vi "rus fit - read freq file.vi"(4 "temperature points IN":dbl[](array[numeric])=array[7043 elements], 5 "right":dbl=10069.29999999702, 6 "time points IN":dbl[](array[numeric])=array[7043 elements], 7 "left":dbl, 8 "file path":path=path "\\\\rus-one\\newdata/data/Ultrasound/Experiment/ProbeTest/Probe10/Hg1201-6-C185-550Cair-3c-83K/sweep3/9w/3366_a.dat", 9 "attenuation points IN":dbl[](array[numeric])=array[7043 elements], 10 "frequency points IN":dbl[](array[numeric])=array[7043 elements], 11 "lorentzian points IN":T1[](array[typedef])=array[7043 elements] {"lorentzian"."z∞ (V)" format="%#_4p"; "lorentzian"."Q" format="%#_4p"; "lorentzian"."φ (rad)" format="%#_3p"; "lorentzian"."Γ (Hz)" format="%#_5p"; "lorentzian"."ω (Hz)" format="%#_9p"; "lorentzian"."A (VHz)" format="%#_3p"}) -> (0 "format version":string="A1", 1 "attenuation points OUT":dbl[](array[numeric]), 2 "frequency points OUT":dbl[](array[numeric]), 3 "lorentzian points OUT":T1[](array[typedef]) {"lorentzian"."z∞ (V)" format="%#_4p"; "lorentzian"."Q" format="%#_4p"; "lorentzian"."φ (rad)" format="%#_3p"; "lorentzian"."Γ (Hz)" format="%#_5p"; "lorentzian"."ω (Hz)" format="%#_9p"; "lorentzian"."A (VHz)" format="%#_3p"})   [LabVIEW 2021]
uses:
  temperature sweep point.ctl
  lorentzian.ctl
  circle corners.ctl
  <vilib>/Utility/file.llb/Read From Spreadsheet File (string).vi
  <vilib>/regexp/Match Regular Expression.xnode
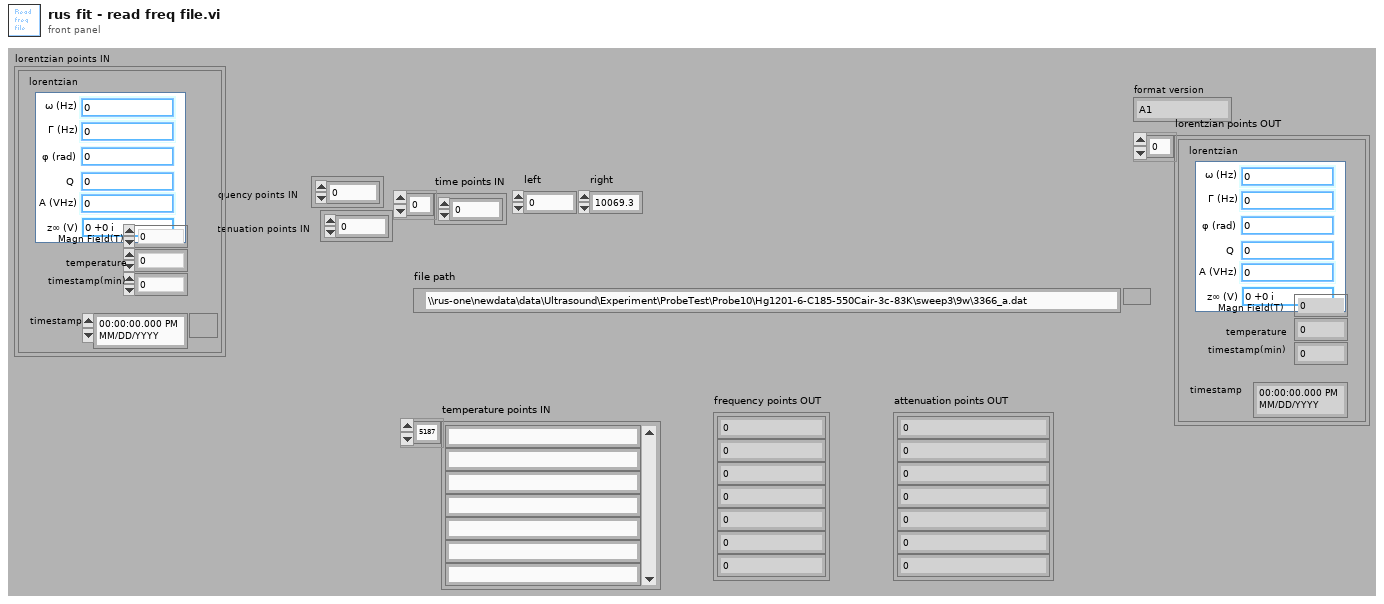
[diagram p1: front panel]
types:
  T1 = typedef "temperature sweep point.ctl" = cluster{"temperature":dbl, "lorentzian":T2, "timestamp(min)":dbl, "timestamp":timestamp, "Magn Field(T)":dbl}
  T2 = typedef "lorentzian.ctl" = cluster{"A (VHz)":dbl, "ω (Hz)":dbl, "Γ (Hz)":dbl, "φ (rad)":dbl, "Q":dbl, "Norm  Ampl":dbl, "z∞ (V)":cdb, "4corners":T3}
  T3 = typedef "circle corners.ctl" = cluster{"z (-pi/2)":cdb, "z(inf)":cdb, "z (pi/2)":cdb, "z center":cdb, "z(0)":cdb, "radius":dbl}
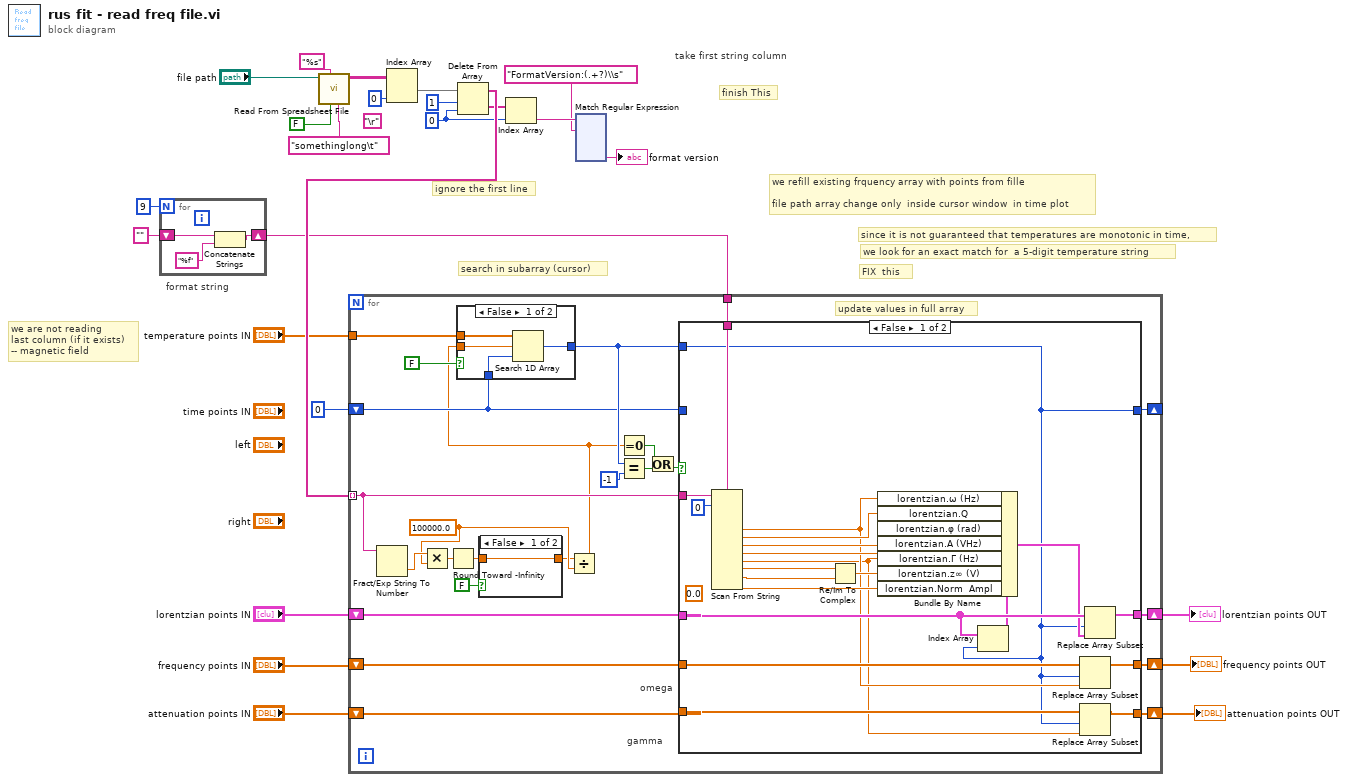
[diagram p0: block diagram]
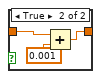
[diagram p2: hidden frame]
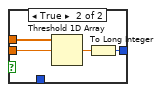
[diagram p3: hidden frame]
diagram:
  w16 = 0 ("index")
  (unwired) "\r"
  # "we are not reading \nlast column (if it exists) \n-- magnetic field"
  # "search in subarray (cursor)"
  # "format string"
  # "since it is not guaranteed that temperatures are monotonic in time,"
  # "we look for an exact match for  a 5-digit temperature string"
  # "FIX  this"
  # "finish This"
  # "take first string column"
  # "we refill existing frquency array with points from fille\n\nfile path array change only  inside cursor window  in time plot"
  # "ignore the first line"
  n1 = for {
    N: 9 -> [_]
    shift-right: [w27] -> w3
    shift-left: "" ("input string") -> [w26]
    n2 = Concatenate Strings(w26, "%f" ("input string")) -> (w27:string)
  }
  n3 = call-poly <vilib>:"Read From Spreadsheet File.vi"("delimiter (\\t)"="somethinglong\t" ("delimiter (\\t)"), "transpose (no:F)"=FALSE ("append to file? (new file:F)"), "format (%s)"="%s", "file path (dialog if empty)"="file path") -> ("all rows"=w22:string[][])  [unwired: 3 in, 4 out]
  n4 = Index Array(array=w22, index (col)=0 ("disabled index (col)")) -> (element=w20:string[])  [unwired: 1 in]
  n5 = Delete From Array(array=w20, length=1, index=w16) -> (deleted portion=w17:string[], array with subset deleted=w18:string[])
  n6 = for {
    shift-right: [w48] -> w9
    shift-left: "attenuation points IN" -> [w47]
    tunnel: w18 -> [w40] mode=indexing
    shift-right: [w51] -> w11
    shift-left: "lorentzian points IN" -> [w52]
    shift-right: [w49] -> w10
    shift-left: "frequency points IN" -> [w50]
    tunnel: "temperature points IN" -> [w41]
    tunnel: w3 -> [w38]
    shift-right: [w37] -> _
    shift-left: 0 -> [w36]
    w33 = 100000.0 ("y")
    # "omega"
    # "gamma"
    # "update values in full array"
    n7 = Fract/Exp String To Number(string=w40) -> (number=w34:dbl)  [unwired: 3 in, 1 out]
    n8 = Multiply(x=w34, y=w33) -> (x*y=w35:dbl)
    n9 = Round Toward -Infinity(1:w35) -> (0:w32:dbl)
    n10 = case shown="False" FALSE {
      tunnel: w32 -> [w53 w55]
      tunnel: [w53 w54] -> w31
      frame False {
      }
      frame True {
        n11 = Add(x=w55, y=0.001) -> (x+y=w54:dbl)
      }
    }
    n12 = Divide(x=w31, y=w33) -> (x/y=w30:dbl)
    n13 = case shown="False" FALSE {
      tunnel: w41 -> [w60 w64]
      tunnel: w30 -> [w59 w61]
      tunnel: [w58 w62] -> w39
      tunnel: w36 -> [w57 _]
      frame False {
        n14 = Search 1D Array(1D array=w60, element=w59, start index (0)=w57) -> (index of element=w58:i32)
      }
      frame True {
        n15 = Threshold 1D Array(2:w61, 3:w64) -> (0:w63:dbl)  [unwired: 1 in]
        n16 = To Long Integer(number=w63) -> (32bit integer=w62:i32)
      }
    }
    n17 = Equal To 0?(x=w30) -> (x = 0?=w46:bool)
    n18 = Equal?(x=w39, y=-1) -> (x = y?=w45:bool)
    n19 = Or(x=w46, y=w45) -> (x .or. y?=w42:bool)
    n20 = case shown="False" w42 {
      tunnel: w52 -> [w80 w89]
      tunnel: [w85 w89] -> w51
      tunnel: w50 -> [w84 w88]
      tunnel: [w83 w88] -> w49
      tunnel: [w82 w87] -> w48
      tunnel: w47 -> [w81 w87]
      tunnel: w39 -> [w65 _]
      tunnel: w38 -> [w71 _]
      tunnel: w40 -> [w70 _]
      tunnel: [w65 w86] -> w37
      tunnel: w36 -> [_ w86]
      frame False {
        (unwired) 0.0 ("default value 10")
        n21 = Scan From String(format string=w71, input string=w70, initial scan location=u32 0) -> (output 2=w67:dbl, output 3=w72:dbl, output 4=w73:dbl, output 5=w74:dbl, output 6=w66:dbl, output 7=w75:dbl, output 8=w76:dbl, output 9=w79:dbl)  [unwired: 11 in, 3 out]
        n22 = Re/Im To Complex(1:w76, 2:w75) -> (0:w78:cdb)
        n23 = Index Array(array=w80, index=w65) -> (element=w69:T1)
        n24 = Bundle By Name(cluster=w69, "lorentzian.ω (Hz)"=w67, "lorentzian.Q"=w72, "lorentzian.φ (rad)"=w73, "lorentzian.A (VHz)"=w74, "lorentzian.Γ (Hz)"=w66, "lorentzian.z∞ (V)"=w78, "lorentzian.Norm  Ampl"=w79) -> (w68:T1)
        n25 = Replace Array Subset(array=w84, new element=w67, index=w65) -> (w83:dbl[])
        n26 = Replace Array Subset(array=w81, new element=w66, index=w65) -> (w82:dbl[])
        n27 = Replace Array Subset(array=w80, new element=w68, index=w65) -> (w85:T1[])
      }
      frame True {
      }
    }
  }
  "lorentzian points OUT" <- w11
  "frequency points OUT" <- w10
  "attenuation points OUT" <- w9
  n28 = Index Array(array=w17, index=w16) -> (element=w15:string)
  n29 = xnode "Match Regular Expression"("input string"=w15, "regular expression"="FormatVersion:(.+?)\\s" ("delimiter (\\t)")) -> ("submatch 1"=→"format version":string)  [unwired: 4 in, 5 out]
